vi "StimFile-Replace Tag.vi"(0 "Params In":T1, 7 "Tag":string, 9 "Value":dbl) -> (4 "Params Out":T1, 15 "error out":errorcluster)   [LabVIEW 2015]
uses:
  StimFile-Params.ctl
  <vilib>/regexp/Match Regular Expression.xnode
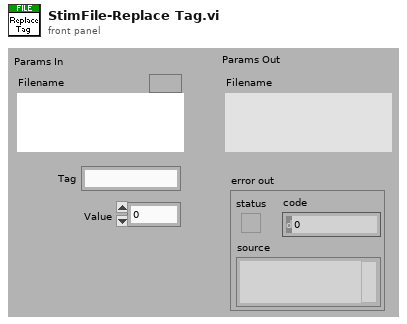
[diagram p1: front panel]
types:
  T1 = typedef "StimFile-Params.ctl" = cluster{"Filename":path, "Signal":dbl[], "Channel":i32, "stream":bool, "offset":i32, "nreps":i32, "loops":i32}
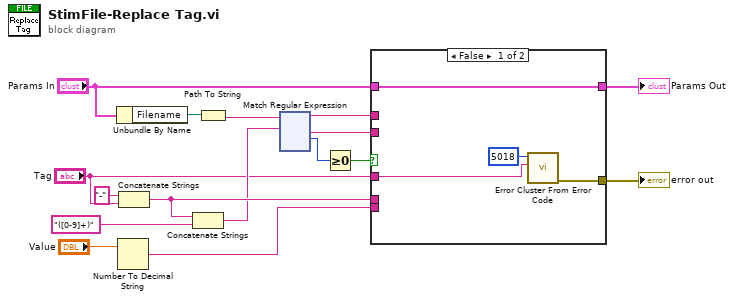
[diagram p0: block diagram]
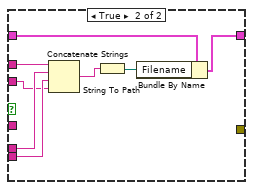
[diagram p2: hidden frame]
diagram:
  n1 = Unbundle By Name("Params In") -> ("Filename"=w16:path)
  n2 = Number To Decimal String(number="Value") -> (decimal integer string=w11:string)  [unwired: 1 in]
  n3 = Concatenate Strings("-" ("string"), "Tag") -> (w13:string)
  n4 = Concatenate Strings(w13, "([0-9]+)" ("string")) -> (w7:string)
  n5 = Path To String(path=w16) -> (string=w8:string)
  n6 = xnode "Match Regular Expression"("input string"=w8, "regular expression"=w7) -> ("before match"=w3:string, "after match"=w4:string, "offset past match"=w6:i32)  [unwired: 4 in, 2 out]
  n7 = Greater Or Equal To 0?(x=w6) -> (x >= 0?=w5:bool)
  n8 = case shown="False" w5 {
    tunnel: w13 -> [_ w28]
    tunnel: w11 -> [_ w27]
    tunnel: "Params In" -> [w20 w26]
    tunnel: [w20 w25] -> w9
    tunnel: w4 -> [_ w22]
    tunnel: w3 -> [_ w23]
    tunnel: "Tag" -> [w18 _]
    tunnel: [w17 _] -> w1
    frame False {
      n9 = call <vilib>:"Error Cluster From Error Code.vi"("error message (\"\")"=w18, "error code (0)"=5018 ("error code (no error:0)")) -> ("error out"=w17:errorcluster)  [unwired: 7 in]
    }
    frame True {
      n10 = Concatenate Strings(w23, w28, w27, w22) -> (w21:string)
      n11 = String To Path(string=w21) -> (path=w24:path)
      n12 = Bundle By Name(cluster=w26, "Filename"=w24) -> (w25:T1)
    }
  }
  "Params Out" <- w9
  "error out" <- w1
